vi "Transcriptor LabVIEW to C code Arduino GUI.vi"(7 "VISA resource name":refnum<visa-resource-name>="COM3", 8 "error in (no error)":errorcluster, 9 "Board type":T1="arduino:avr:nano", 10 "Arduino IDE installation directory":path=path "c:/Program Files/Arduino/arduino.exe ", 11 "vi path":path) -> (0 "error out":errorcluster, 1 "transcripted code":string, 2 "standard error":string, 3 "standard output":string)   [LabVIEW 2014]
uses:
  types/LabVIEW Universal Transcriptor Arduino Boards Specific Names.ctl
panel:
  in  "Defines":string[](array[string])=["using namespace std;"]
  in  "Includes":string[](array[string])=["<ArduinoSTL.h>", "<vector>"]
  # "Use Arduino.h just for arduino\nNO for ESP8266!"
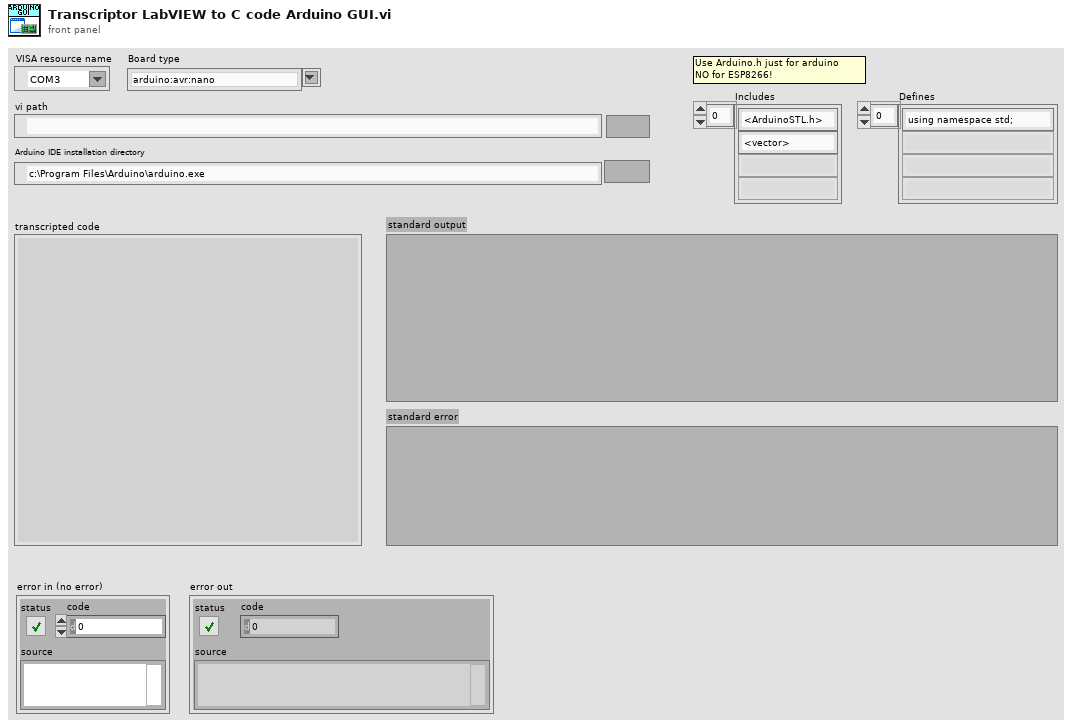
[diagram p1: front panel]
types:
  T1 = typedef "LabVIEW Universal Transcriptor Arduino Boards Specific Names.ctl" = string
  T2 = enum16{"open", "replace", "create", "open or create", "replace or create", "replace or create with confirmation"}
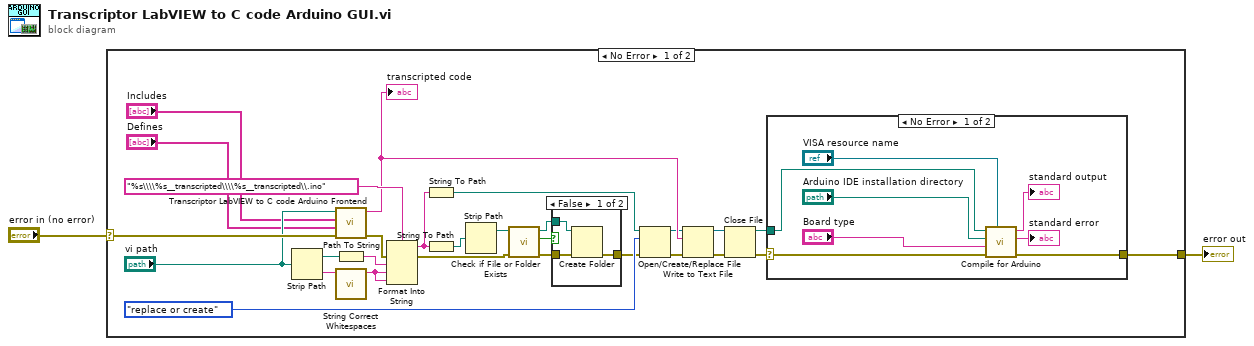
[diagram p0: block diagram]
diagram:
  n1 = case shown="No Error" "error in (no error)" {
    selector: "error in (no error)" -> [w30 w44]
    tunnel: [w5 w44] -> w1
    frame No Error {
      n2 = Strip Path(path="vi path") -> (stripped path=w25:path, name=w28:string)
      n3 = call "Transcriptor LabVIEW to C code Arduino Frontend.vi"("error in"=w30, "Defines"="Defines", "Includes"="Includes", "vi path"="vi path") -> ("error out"=w27:errorcluster, "transcripted code"=w23:string)  [unwired: 6 in]
      "transcripted code" <- w23
      n4 = Path To String(path=w25) -> (string=w24:string)
      n5 = call "String Correct Whitespaces.vi"("String in"=w28) -> ("String out"=w13:string)  [unwired: 10 in]
      n6 = Format Into String(format string="%s\\\\%s__transcripted\\\\%s__transcripted\\.ino", error in=w27, w24, w13, w13) -> (resulting string=w14:string, error out=w12:errorcluster)  [unwired: 1 in]
      n7 = String To Path(string=w14) -> (path=w19:path)
      n8 = String To Path(string=w14) -> (path=w15:path)
      n9 = Strip Path(path=w15) -> (stripped path=w10:path)  [unwired: 1 out]
      n10 = call <vilib>:"Check if File or Folder Exists.vi"("error in (no error)"=w12, "path"=w10) -> ("error out"=w11:errorcluster, "file or folder exists?"=w9:bool, "dup path"=w8:path)  [unwired: 7 in]
      n11 = case shown="False" w9 {
        tunnel: [w42 w43] -> w16
        tunnel: w11 -> [w41 w43]
        tunnel: w8 -> [w40 _]
        frame False {
          n12 = Create Folder(path (use dialog)=w40, error in=w41) -> (error out=w42:errorcluster)  [unwired: 1 in, 2 out]
        }
        frame True {
        }
      }
      n13 = Open/Create/Replace File(file path (use dialog)=w19, error in=w16, operation (0:open)=T2."replace or create") -> (refnum out=w17:refnum<file>, error out=w20:errorcluster)  [unwired: 3 in, 1 out]
      n14 = Write to Text File(file (use dialog)=w17, text=w23, error in=w20) -> (refnum out=w21:refnum<file>, error out=w22:errorcluster)  [unwired: 1 in, 1 out]
      n15 = Close File(refnum=w21, error in=w22) -> (path=w6:path, error out=w7:errorcluster)
      n16 = case shown="No Error" w7 {
        selector: w7 -> [w38 w39]
        tunnel: w6 -> [w36 _]
        tunnel: [w37 w39] -> w5
        frame No Error {
          n17 = call "Compile for Arduino.vi"("VISA resource name"="VISA resource name", "Error In"=w38, "Combo Box"="Board type", "Arduino IDE installation directory"="Arduino IDE installation directory", "input filename"=w36) -> ("Error Out"=w37:errorcluster, "standard error"=→"standard error":string, "standard output"=→"standard output":string)  [unwired: 4 in]
        }
        frame Error {
        }
      }
    }
    frame Error {
    }
  }
  "error out" <- w1
